vi "Clear Errors from Array.vi"(8 "Error In":errorcluster, 11 "Errors to clear":errorcluster[](array[cluster])) -> (0 "Error Out":errorcluster, 3 "specific error cleared?":bool)   [LabVIEW 2015]
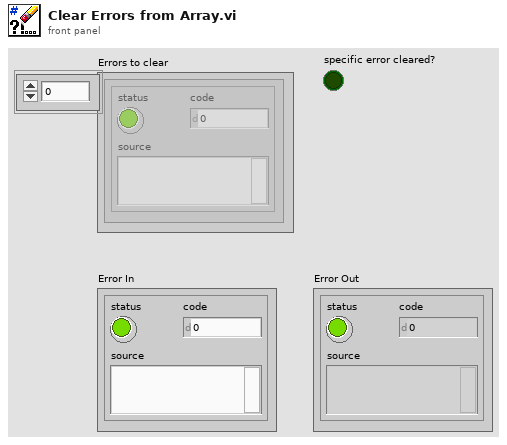
[diagram p1: front panel]
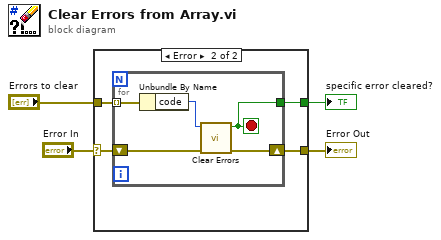
[diagram p0: block diagram]
diagram:
  n1 = case shown="Error" "Error In" {
    selector: "Error In" -> [w5 w7]
    tunnel: "Errors to clear" -> [_ w9]
    tunnel: [w5 w8] -> w3
    tunnel: [_ w6] -> w1
    frame No Error {
    }
    frame Error {
      n2 = for {
        tunnel: w9 -> [w14] mode=indexing
        shift-right: [w11] -> w8
        shift-left: w7 -> [w12]
        tunnel: [w10] -> w6
        stop <- w10 stop-if-true
        n3 = Unbundle By Name(w14) -> ("code"=w13:i32)
        n4 = call <vilib>:"Clear Errors.vi"("error in (no error)"=w12, "specific error code to clear (0: all)"=w13) -> ("error out"=w11:errorcluster, "specific error cleared?"=w10:bool)  [unwired: 4 in]
      }
    }
  }
  "Error Out" <- w3
  "specific error cleared?" <- w1
